vi "UDP add last update channel test.vi"() -> (0 "error out":errorcluster, 3 "UDP Last Update Channel Success":bool)   [LabVIEW 2015, in "E2E Tag Exchange tests.lvlib"]
uses:
  E2E Tag Exchange tests.lvlib
  module/configuration/Runtime Implementation.ctl
  <vilib>/NI/Tag Bus/tag/Data Type.ctl
  <vilib>/NI/Tag Bus Module Framework/channel/channel classification.ctl
  module/configuration/E2E Tag Exchange configuration.lvclass/E2E Tag Exchange configuration.ctl
  <vilib>/NI/Tag Bus Module Framework/channel/TBM channel.lvclass
  module/configuration/E2E Tag Exchange configuration.lvclass
  <vilib>/NI/Tag Bus/tag/tag descriptor.lvclass
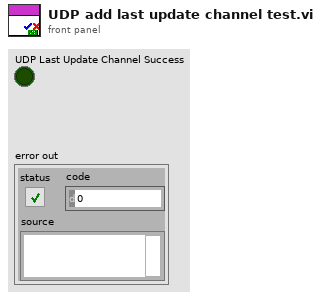
[diagram p1: front panel]
types:
  T1 = typedef "TBM channel.lvclass/channel classification.ctl" = enum16{"input data", "output data", "processing parameter", "processing result"}
  T2 = typedef "tag bus.lvlib/tag descriptor.lvclass/Data Type.ctl" = enum16{"Double", "Single", "I64", "I32", "I16", "I8", "U64", "U32", "U16", "U8", "Boolean", "String", "Array of Double", "Array of Single", "Array of I64", "Array of I32", "Array of I16", "Array of I8", "Array of U64", "Array of U32", "Array of U16", "Array of U8", "Array of Boolean", "Array of String"}
  T3 = typedef "E2E Tag Exchange configuration.lvclass/Runtime Implementation.ctl" = enum16{"RT FIFO", "UDP"}
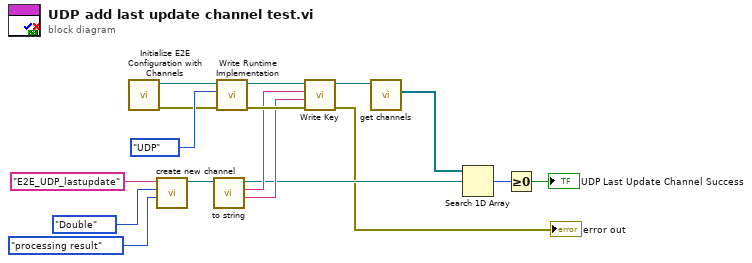
[diagram p0: block diagram]
diagram:
  n1 = call "Initialize E2E Configuration with Channels.vi"() -> ("error out"=w7:errorcluster, "Initialized E2E configuration"=w8:refnum<class "E2E Tag Exchange configuration.lvclass">)  [unwired: 9 in, 1 out]
  n2 = call <vilib>:"create new channel.vi"("channel classification"=channel_classification."processing result", "data type"=Data_Type."Double", "channel name"="E2E_UDP_lastupdate" ("Key")) -> ("channel"=w14:refnum<class "TBM channel.lvclass">)  [unwired: 8 in]
  n3 = call-dynamic "to string.vi"("channel in"=w14) -> ("channel data"=w9:string, "identifier"=w10:string, "channel out"=w4:refnum<class "TBM channel.lvclass">)  [unwired: 7 in, 1 out]
  n4 = call "Write Runtime Implementation.vi"("error in (no error)"=w7, "Runtime Implementation"=Runtime_Implementation."UDP", "E2E Tag Exchange configuration in"=w8) -> ("error out"=w13:errorcluster, "E2E Tag Exchange configuration out"=w11:refnum<class "E2E Tag Exchange configuration.lvclass">)  [unwired: 7 in]
  n5 = call "Write Key.vi"("error in"=w13, "Value"=w9, "Key"=w10, "E2E configuration in"=w11) -> ("error out"=→"error out":errorcluster, "E2E configuration out"=w6:refnum<class "E2E Tag Exchange configuration.lvclass">)  [unwired: 6 in]
  n6 = call-dynamic "get channels.vi"("E2E configuration in"=w6) -> ("channels"=w5:refnum<class "TBM channel.lvclass">[])  [unwired: 9 in, 1 out]
  n7 = Search 1D Array(1D array=w5, element=w4) -> (index of element=w3:i32)  [unwired: 1 in]
  n8 = Greater Or Equal To 0?(x=w3) -> (x >= 0?=→"UDP Last Update Channel Success":bool)
